vi "Inflation Camera - Screen Grab.vi"(8 "error in (no error)":errorcluster, 9 "gui notifier":refnum<notifier>, 10 "error queue":refnum<queue>, 11 "cam notifier":refnum<notifier>) -> (0 "error out":errorcluster)   [LabVIEW 2020]
uses:
  Hardware/Sensors/Cameras/Camera.lvclass
  Main GUI Loop/Handler.ctl
  Hardware/Sensors/Cameras/Camera.lvclass/Camera.ctl
panel:
  out "current image":T1(plugin-control)
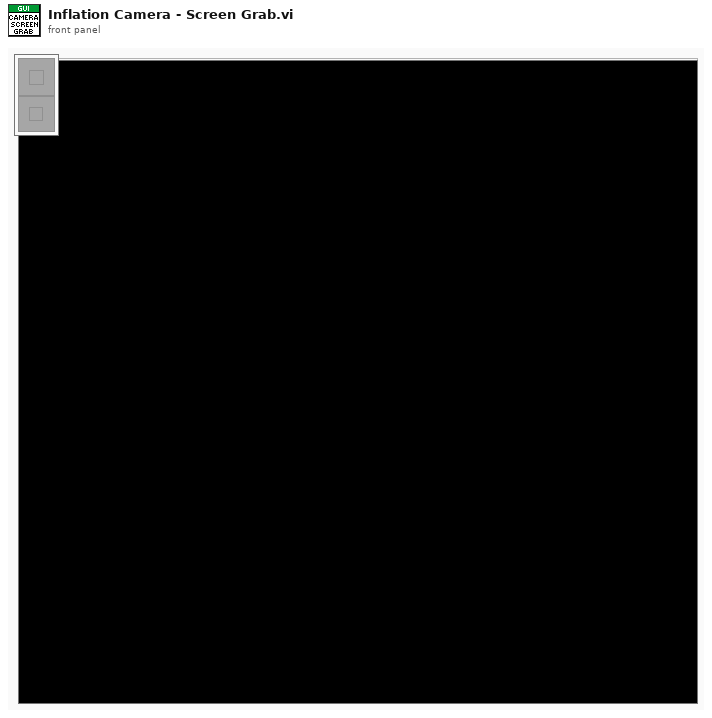
[diagram p1: front panel]
types:
  T1 = typedef "IMAQ Image.ctl" = refnum<image>
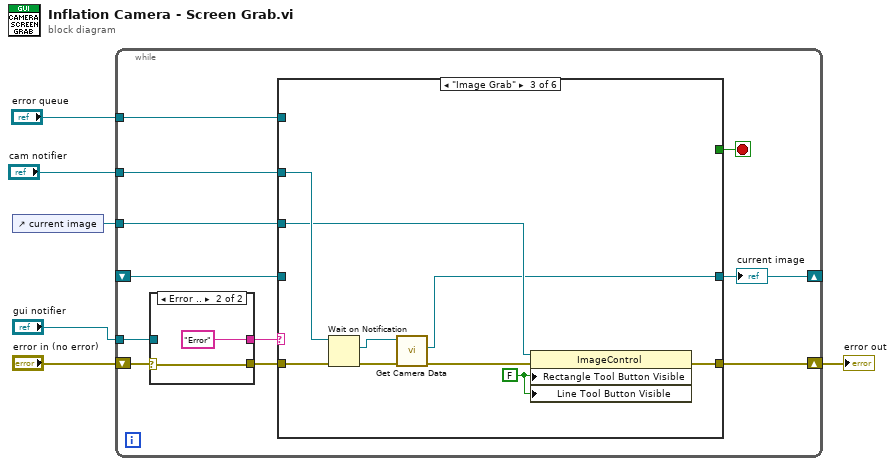
[diagram p0: block diagram]
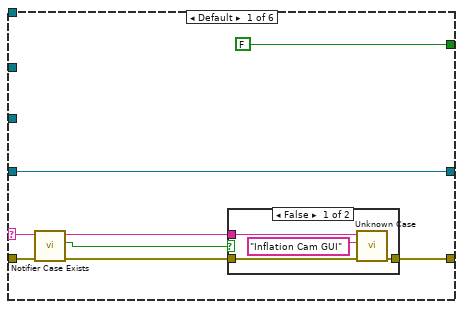
[diagram p2: hidden frame]
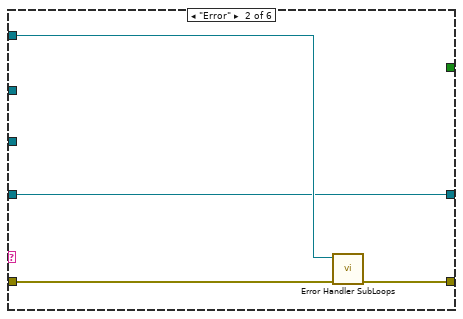
[diagram p4: hidden frame]
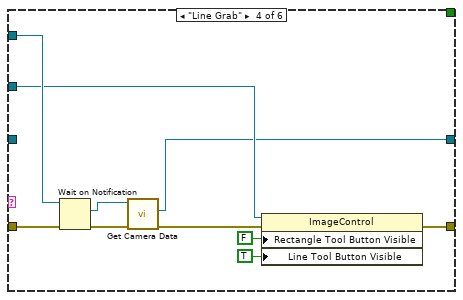
[diagram p5: hidden frame]
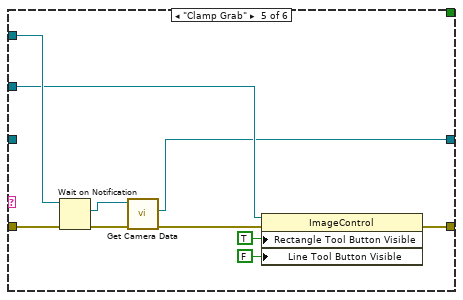
[diagram p6: hidden frame]
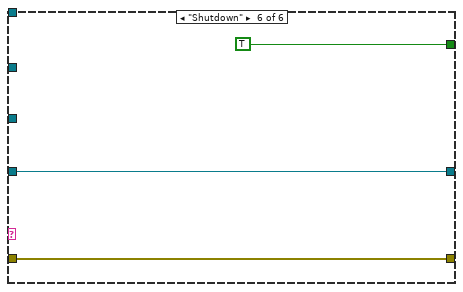
[diagram p7: hidden frame]
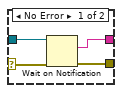
[diagram p8: hidden frame]
diagram:
  n1 = control-ref of="current image"() -> (w1:refnum<vi>)
  n2 = while {
    tunnel: "cam notifier" -> [w16]
    tunnel: "gui notifier" -> [w15]
    shift-right: [w12] -> w3
    shift-left: "error in (no error)" -> [w14]
    tunnel: "error queue" -> [w10]
    tunnel: w1 -> [w9]
    shift-right: [w8] -> _
    shift-left: _ -> [w7]
    stop <- w17 stop-if-true
    n3 = case shown="Error .." w14 {
      selector: w14 -> [w68 w72]
      tunnel: w15 -> [w70 _]
      tunnel: [w69 w72] -> w13
      tunnel: [w67 "Error" ("gui msg")] -> w11
      frame No Error {
        n4 = Wait on Notification(notifier=w70, error in (no error)=w68) -> (notification=w67:string, error out=w69:errorcluster)  [unwired: 2 in, 2 out]
      }
      frame Error {
      }
    }
    n5 = case shown="\"Image Grab\"" w11 {
      selector: w11 -> [w23 _ _ _ _ _]
      tunnel: [FALSE _ _ _ _ TRUE] -> w17
      tunnel: w16 -> [_ _ w41 w51 w61 _]
      tunnel: w13 -> [w22 w33 w40 w50 w60 w65]
      tunnel: [w24 w32 w36 w46 w56 w65] -> w12
      tunnel: w10 -> [_ w34 _ _ _ _]
      tunnel: w9 -> [_ _ w39 w49 w59 _]
      tunnel: [w18 w31 w35 w45 w55 w64] -> w8
      tunnel: w7 -> [w18 w31 _ _ _ w64]
      frame Default {
        n6 = call "Notifier Case Exists.vi"("error in (no error)"=w22, "case in"=w23) -> ("error out"=w21:errorcluster, "defined case?"=w20:bool, "case out"=w19:string)  [unwired: 7 in]
        n7 = case shown="False" w20 {
          tunnel: w21 -> [w29 w30]
          tunnel: [w28 w30] -> w24
          tunnel: w19 -> [w26 _]
          frame False {
            n8 = call "Unknown Case.vi"("error in (no error)"=w29, "source"="Inflation Cam GUI", "case"=w26) -> ("error out"=w28:errorcluster)  [unwired: 8 in]
          }
          frame True {
          }
        }
      }
      frame "Error" {
        n9 = call "Error Handler SubLoops.vi"("error in"=w33, "main gui queue"=w34) -> ("error out"=w32:errorcluster)  [unwired: 9 in]
      }
      frame "Image Grab" {
        w38 = FALSE ("ROI Tool Buttons Visible:Rectangle Tool Button Visible")
        n10 = Wait on Notification(notifier=w41, error in (no error)=w40) -> (notification=w43:refnum<class "Camera.lvclass">, error out=w42:errorcluster)  [unwired: 2 in, 2 out]
        n11 = call "Get Camera Data.vi"("error in (no error)"=w42, "Camera in"=w43) -> ("error out"=w37:errorcluster, "image"=w35:T1)  [unwired: 5 in, 3 out]
        n12 = property class="ImageControl"(reference=w39, error in=w37, "Rectangle Tool Button Visible"=w38, "Line Tool Button Visible"=w38) -> (error out=w36:errorcluster)  [unwired: 1 out]
      }
      frame "Line Grab" {
        n13 = Wait on Notification(notifier=w51, error in (no error)=w50) -> (notification=w53:refnum<class "Camera.lvclass">, error out=w52:errorcluster)  [unwired: 2 in, 2 out]
        n14 = call "Get Camera Data.vi"("error in (no error)"=w52, "Camera in"=w53) -> ("error out"=w47:errorcluster, "image"=w45:T1)  [unwired: 5 in, 3 out]
        n15 = property class="ImageControl"(reference=w49, error in=w47, "Rectangle Tool Button Visible"=FALSE ("ROI Tool Buttons Visible:Rectangle Tool Button Visible"), "Line Tool Button Visible"=TRUE ("ROI Tool Buttons Visible:Line Tool Button Visible")) -> (error out=w46:errorcluster)  [unwired: 1 out]
      }
      frame "Clamp Grab" {
        n16 = Wait on Notification(notifier=w61, error in (no error)=w60) -> (notification=w63:refnum<class "Camera.lvclass">, error out=w62:errorcluster)  [unwired: 2 in, 2 out]
        n17 = call "Get Camera Data.vi"("error in (no error)"=w62, "Camera in"=w63) -> ("error out"=w57:errorcluster, "image"=w55:T1)  [unwired: 5 in, 3 out]
        n18 = property class="ImageControl"(reference=w59, error in=w57, "Rectangle Tool Button Visible"=TRUE ("ROI Tool Buttons Visible:Rectangle Tool Button Visible"), "Line Tool Button Visible"=FALSE ("ROI Tool Buttons Visible:Line Tool Button Visible")) -> (error out=w56:errorcluster)  [unwired: 1 out]
      }
      frame "Shutdown" {
      }
    }
    "current image" <- w8
  }
  "error out" <- w3
